vi "WiringPi_PWMWrite.vi"(7 "Value":u16, 8 "error in (no error)":errorcluster, 11 "WiringPi GPIO":T1=7 items=["Pin1_3.3V"=51, "Pin2_5V"=52, "Pin3_GPIO8_I2C1_SDA"=8, "Pin4_5V"=53, "Pin5_GPIO9_I2C1_SCL"=9, "Pin6_Gnd"=54, "Pin7_GPIO7_GPCLK0"=7, "Pin8_GPIO15_TXD_UART"=15, "Pin9_Gnd"=55, "Pin10_GPIO16_RXD_UART"=16, "Pin11_GPIO0"=0, "Pin12_GPIO1_PCMCLK_PWM0"=1, "Pin13_GPIO2"=2, "Pin14_Gnd"=56, "Pin15_GPIO3"=3, "Pin16_GPIO4"=4, "Pin17_3V"=57, "Pin18_GPIO5"=5, "Pin19_GPIO12_MOSI(SPI)"=12, "Pin20_Gnd"=58, "Pin21_GPIO13_MISO(SPI)"=13, "Pin22_GPIO6"=6, "Pin23_GPIO14_CLK(SPI)"=14, "Pin24_GPIO10_CE0_SPI"=10, "Pin25_Gnd"=59, "Pin26_GPIO11_CE1_SPI"=11, "Pin27_SDA0_I2C_EEPROM"=60, "Pin28_SCL0_I2C_EEPROM"=61, "Pin_29_GPIO21_GPCLK1"=21, "Pin30_Gnd"=62, "Pin31_GPIO22_GPCLK2"=22, "Pin32_GPIO26_PWM0"=26, "Pin33_GPIO23_PWM1"=23, "Pin34_Gnd"=63, "Pin35_GPIO24_PCMFS_PWM1"=24, "Pin36_GPIO27"=27, "Pin37_GPIO25"=25, "Pin38_GPIO28_PCM_DIN"=28, "Pin39_Gnd"=64, "Pin40_GPIO29_PCM_DOUT"=29]) -> (0 "error out":errorcluster)   [LabVIEW 2014, in "QwaveSys RPi Training Library.lvlib"]
uses:
  <vilib>/Q-Wave Systems/QwaveSys RPi Package 2.0/Addons/QwaveSys RPi Training Library.lvlib
  <vilib>/Q-Wave Systems/QwaveSys RPi Package 2.0/Addons/WiringPi/WiringPi GPIO TypeDef.ctl
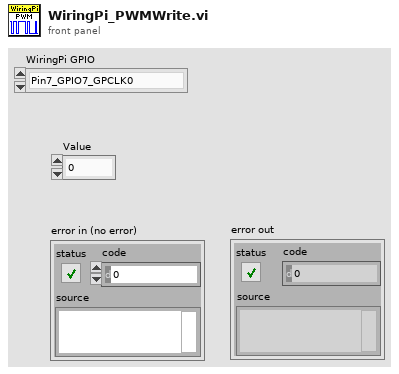
[diagram p1: front panel]
types:
  T1 = typedef "QwaveSys RPi Training Library.lvlib/WiringPi GPIO TypeDef.ctl" = u8
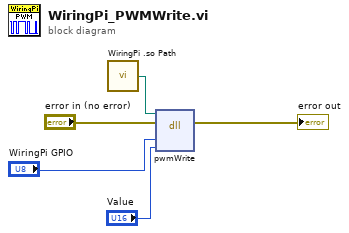
[diagram p0: block diagram]
diagram:
  n1 = call <vilib>:"WiringPi .so Path.vi"() -> ("WiringPi .so Path"=w2:path)  [unwired: 5 in]
  n2 = dll-call lib="libwiringPi.so" fn="pwmWrite"(path in=w2, error in="error in (no error)", "pin"="WiringPi GPIO", "value"="Value") -> (error out=→"error out":errorcluster)  [unwired: 4 in, 1 out]
